vi "Pause While Loop During Execution_LV2012_NI Verified.vi"() -> ()   [LabVIEW 2021]
doc: "This example demonstrates how to pause a while loop using local variables."
panel:
  out "Iteration":i32
  in  "stop":bool
  # "Overview: This example demonstrates how to pause a while loop using local variables.\nRequirements: LabVIEW 2012 (or compatible)\nInstructions:\n1. Run the VI\n2. Click on Pause/Continue to suspend execution\n3. Click on Pause/Continue again to continue executing\n4. Stop the program"
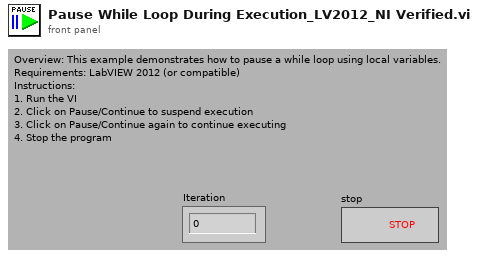
[diagram p1: front panel]
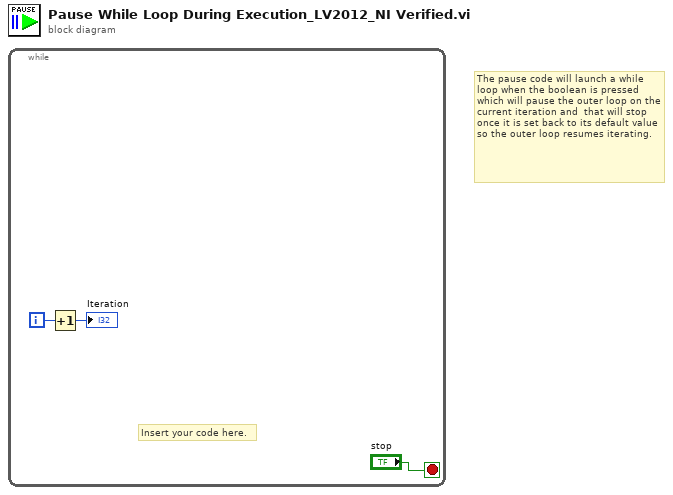
[diagram p0: block diagram]
diagram:
  # "The pause code will launch a while loop when the boolean is pressed which will pause the outer loop on the current iteration and  that will stop once it is set back to its default value so the outer loop resumes iterating."
  n1 = while {
    i -> [w1]
    stop <- "stop" stop-if-true
    # "Insert your code here."
    n2 = Increment(x=w1) -> (x+1=→"Iteration":i32)
  }
